vi "Returning Values By Reference String.vi"(10 "newString":string, 11 "str":string) -> (2 "newString out":string, 3 "str out":string)   [LabVIEW 2018, in "ParsingDataSampleDLL.lvlib"]
doc: "__declspec(dllexport) void ReturningValuesByReference_String (char *str, char **newString);"
uses:
  ParsingDataSampleDLL.lvlib
  ni_reference_vs/Debug/ParsingDataSampleDLL.dll
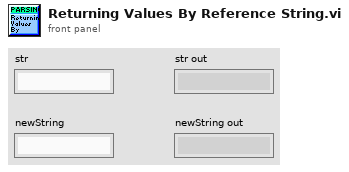
[diagram p1: front panel]
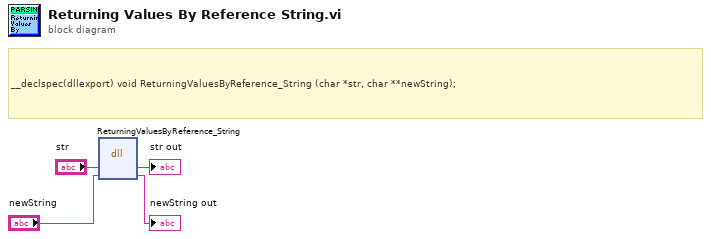
[diagram p0: block diagram]
diagram:
  # "__declspec(dllexport) void ReturningValuesByReference_String (char *str, char **newString);"
  n1 = dll-call lib="C:/Users/celit/Documents/GitHub/Labview_Python_DLL_Call/ni_reference_vs/Debug/ParsingDataSampleDLL.*" fn="ReturningValuesByReference_String"("str"="str", "newString"="newString") -> ("str"=→"str out":string, "newString"=→"newString out":string)  [unwired: 4 in, 2 out]
